vi "Set Config and Get Current.vi"(0 "PowerSupply_IT6333A in":refnum<class "PowerSupply_IT6333A.lvclass">, 5 "CMD":u16(ring)=49408 items=["CH1 OUT OFF"=49408, "CH1 OUT ON"=49409, "CH2 OUT OFF"=49664, "CH2 OUT ON"=49665, "CH3 OUT OFF"=49920, "CH3 OUT ON"=49921, "CH1 OUT Current"=49410, "CH2 OUT Current"=49666, "CH3 OUT Current"=49922, "CH1 Set MAX Current"=49411, "CH2 Set MAX Current"=49667, "CH3 Set MAX Current"=49923], 7 "Voltage(V)":string="0V", 9 "MAX Current(A)":string="1A", 11 "error in (no error)":errorcluster) -> (4 "PowerSupply_IT6333A out":refnum<class "PowerSupply_IT6333A.lvclass">, 6 "read buffer":string, 8 "Current Value":dbl, 15 "error out":errorcluster)   [LabVIEW 2017, in "PowerSupply_IT6333A.lvclass"]
uses:
  PowerSupply_IT6333A.lvclass
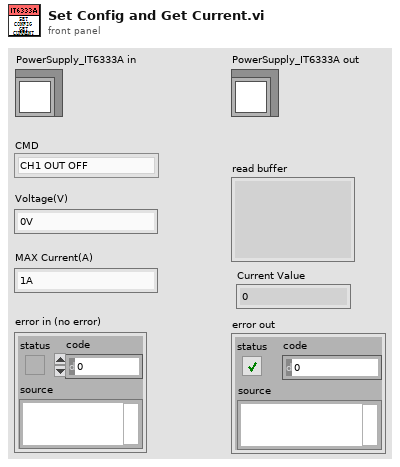
[diagram p1: front panel]
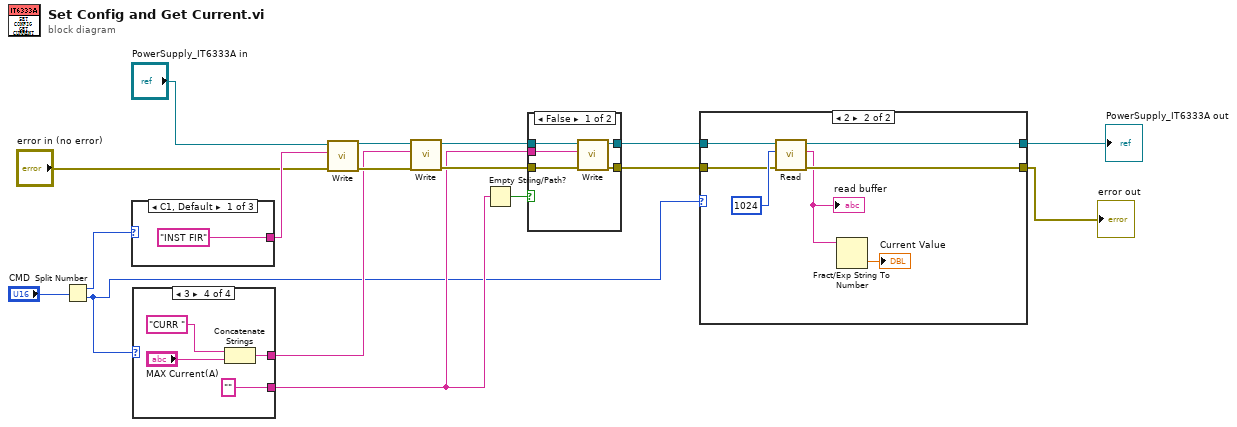
[diagram p0: block diagram]
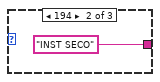
[diagram p4: hidden frame]
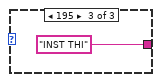
[diagram p5: hidden frame]
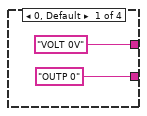
[diagram p6: hidden frame]
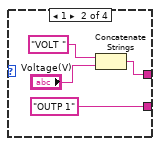
[diagram p7: hidden frame]
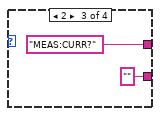
[diagram p8: hidden frame]
diagram:
  n1 = Split Number(x="CMD") -> (hi(x)=w14:u8, lo(x)=w5:u8)
  n2 = case shown="C1, Default" w14 {
    tunnel: ["INST FIR" "INST SECO" "INST THI"] -> w13
    frame 193, Default {
    }
    frame 194 {
    }
    frame 195 {
    }
  }
  n3 = case shown="3" w5 {
    tunnel: ["OUTP 0" "OUTP 1" "" ""] -> w7
    tunnel: ["VOLT 0V" w23 "MEAS:CURR?" w30] -> w10
    frame 0, Default {
    }
    frame 1 {
      n4 = Concatenate Strings("VOLT ", "Voltage(V)") -> (w23:string)
    }
    frame 2 {
    }
    frame 3 {
      n5 = Concatenate Strings("CURR ", "MAX Current(A)") -> (w30:string)
    }
  }
  n6 = call-dynamic "Write.vi"("error in (no error)"="error in (no error)", "write visa cmd buffer"=w13, "PowerSupply_IT6333A in"="PowerSupply_IT6333A in") -> ("error out"=w16:errorcluster, "PowerSupply_IT6333A out"=w17:refnum<class "PowerSupply_IT6333A.lvclass">)  [unwired: 7 in]
  n7 = call-dynamic "Write.vi"("error in (no error)"=w16, "write visa cmd buffer"=w10, "PowerSupply_IT6333A in"=w17) -> ("error out"=w11:errorcluster, "PowerSupply_IT6333A out"=w12:refnum<class "PowerSupply_IT6333A.lvclass">)  [unwired: 7 in]
  n8 = Empty String/Path?(string/path=w7) -> (empty?=w6:bool)
  n9 = case shown="False" w6 {
    tunnel: w12 -> [w37 w39]
    tunnel: w11 -> [w36 w38]
    tunnel: w7 -> [w35 _]
    tunnel: [w34 w38] -> w9
    tunnel: [w33 w39] -> w8
    frame False {
      n10 = call-dynamic "Write.vi"("error in (no error)"=w36, "write visa cmd buffer"=w35, "PowerSupply_IT6333A in"=w37) -> ("error out"=w34:errorcluster, "PowerSupply_IT6333A out"=w33:refnum<class "PowerSupply_IT6333A.lvclass">)  [unwired: 7 in]
    }
    frame True {
    }
  }
  n11 = case shown="2" w5 {
    tunnel: [w40 w48] -> w3
    tunnel: [w41 w47] -> w4
    tunnel: w9 -> [w40 w45]
    tunnel: w8 -> [w41 w44]
    frame 0, Default {
    }
    frame 2 {
      n12 = call-dynamic "Read.vi"("error in (no error)"=w45, "byte count"=u32 1024, "PowerSupply_IT6333A in"=w44) -> ("error out"=w48:errorcluster, "read buffer"=w43:string, "PowerSupply_IT6333A out"=w47:refnum<class "PowerSupply_IT6333A.lvclass">)  [unwired: 6 in]
      "read buffer" <- w43
      n13 = Fract/Exp String To Number(string=w43) -> (number=→"Current Value":dbl)  [unwired: 3 in, 1 out]
    }
  }
  "PowerSupply_IT6333A out" <- w4
  "error out" <- w3
